vi "Ritter STP Correction.vi"(7 "Meter Type":enum16{"Dry Meter", "Wet Meter"}(ring)=enum."Wet Meter", 8 "error in":errorcluster, 10 "Inficon Data Output":T2, 11 "Ritter Data":T1) -> (0 "error out":errorcluster, 3 "Ritter Data Output":T1)   [LabVIEW 2023]
uses:
  Drivers/Ritter Gas Meter/Type Definitions/Ritter Data.ctl
  Drivers/Inficon Fusion Micro GC/Type Definitions/Inficon Data.ctl
panel:
  # "Natural Gas"
  # "Propane"
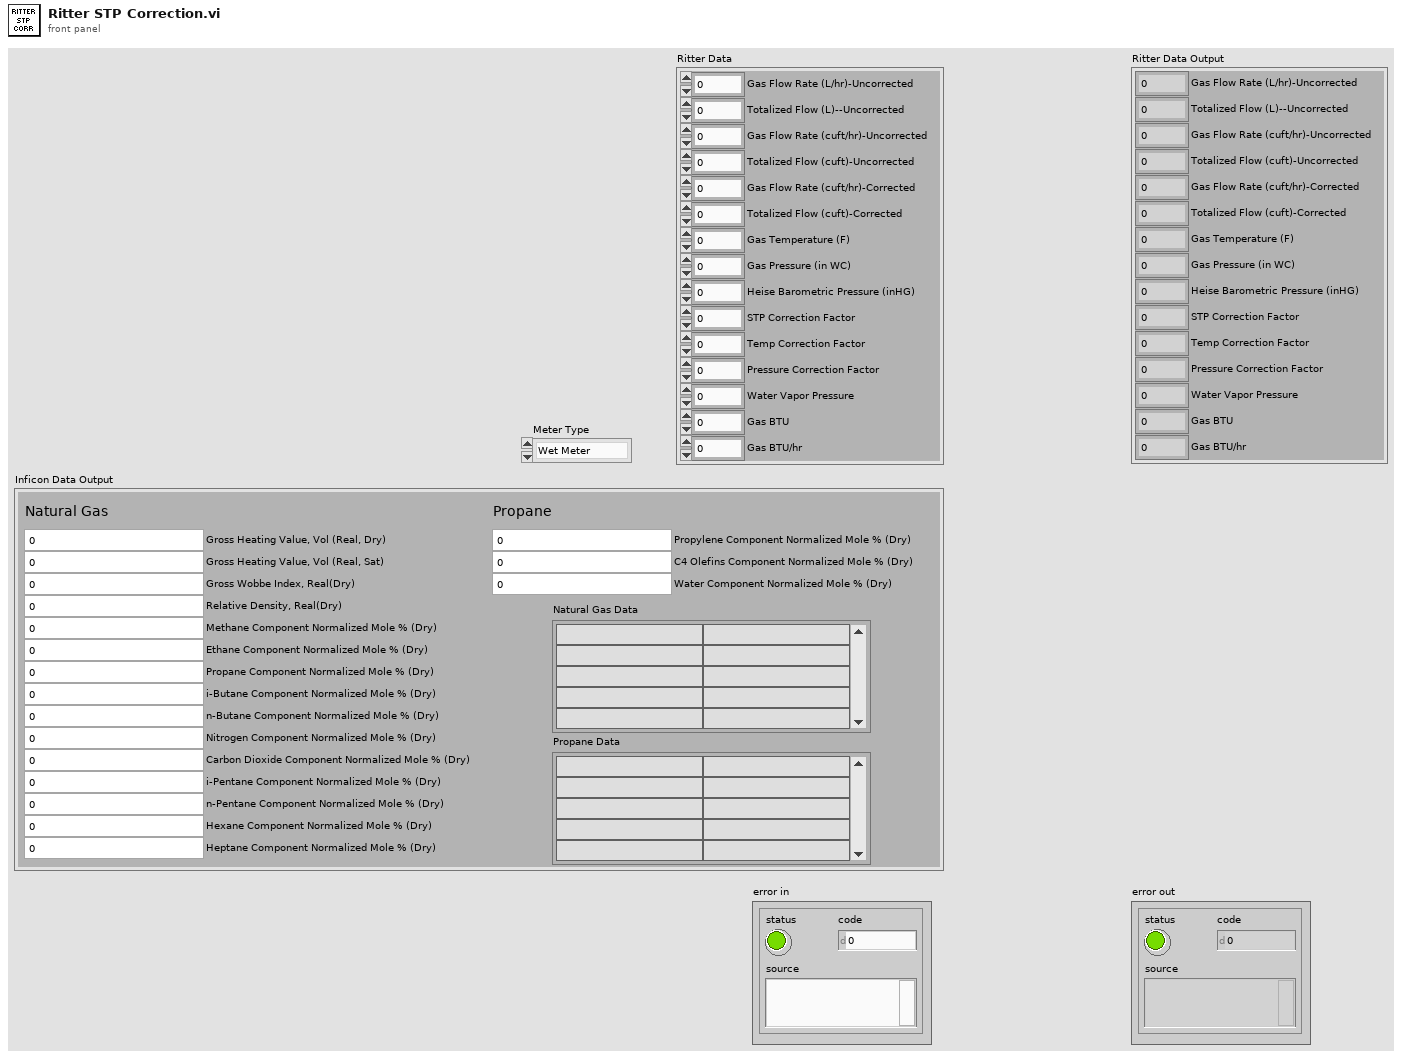
[diagram p1: front panel]
types:
  T1 = typedef "Ritter Data.ctl" = cluster{"Gas Flow Rate (L/hr)-Uncorrected":dbl, "Totalized Flow (L)--Uncorrected":dbl, "Gas Flow Rate (cuft/hr)-Uncorrected":dbl, "Totalized Flow (cuft)-Uncorrected":dbl, "Gas Temperature (F)":dbl, "Gas Pressure (in WC)":dbl, "Heise Barometric Pressure (inHG)":dbl, "STP Correction Factor":dbl, "Temp Correction Factor":dbl, "Pressure Correction Factor":dbl, "Water Vapor Pressure":dbl, "Gas Flow Rate (cuft/hr)-Corrected":dbl, "Totalized Flow (cuft)-Corrected":dbl, "Gas BTU":dbl, "Gas BTU/hr":dbl}
  T2 = typedef "Inficon Data.ctl" = cluster{"Gross Heating Value, Vol (Real, Dry)":dbl, "Nitrogen Component Normalized Mole % (Dry)":dbl, "Methane Component Normalized Mole % (Dry)":dbl, "Carbon Dioxide Component Normalized Mole % (Dry)":dbl, "Ethane Component Normalized Mole % (Dry)":dbl, "Propane Component Normalized Mole % (Dry)":dbl, "i-Pentane Component Normalized Mole % (Dry)":dbl, "i-Butane Component Normalized Mole % (Dry)":dbl, "n-Butane Component Normalized Mole % (Dry)":dbl, "n-Pentane Component Normalized Mole % (Dry)":dbl, "Hexane Component Normalized Mole % (Dry)":dbl, "Heptane Component Normalized Mole % (Dry)":dbl, "Gross Wobbe Index, Real(Dry)":dbl, "Relative Density, Real(Dry)":dbl, "Propylene Component Normalized Mole % (Dry)":dbl, "C4 Olefins Component Normalized Mole % (Dry)":dbl, "Water Component Normalized Mole % (Dry)":dbl, "Gross Heating Value, Vol (Real, Sat)":dbl, "Natural Gas Data":string[][], "Propane Data":string[][]}
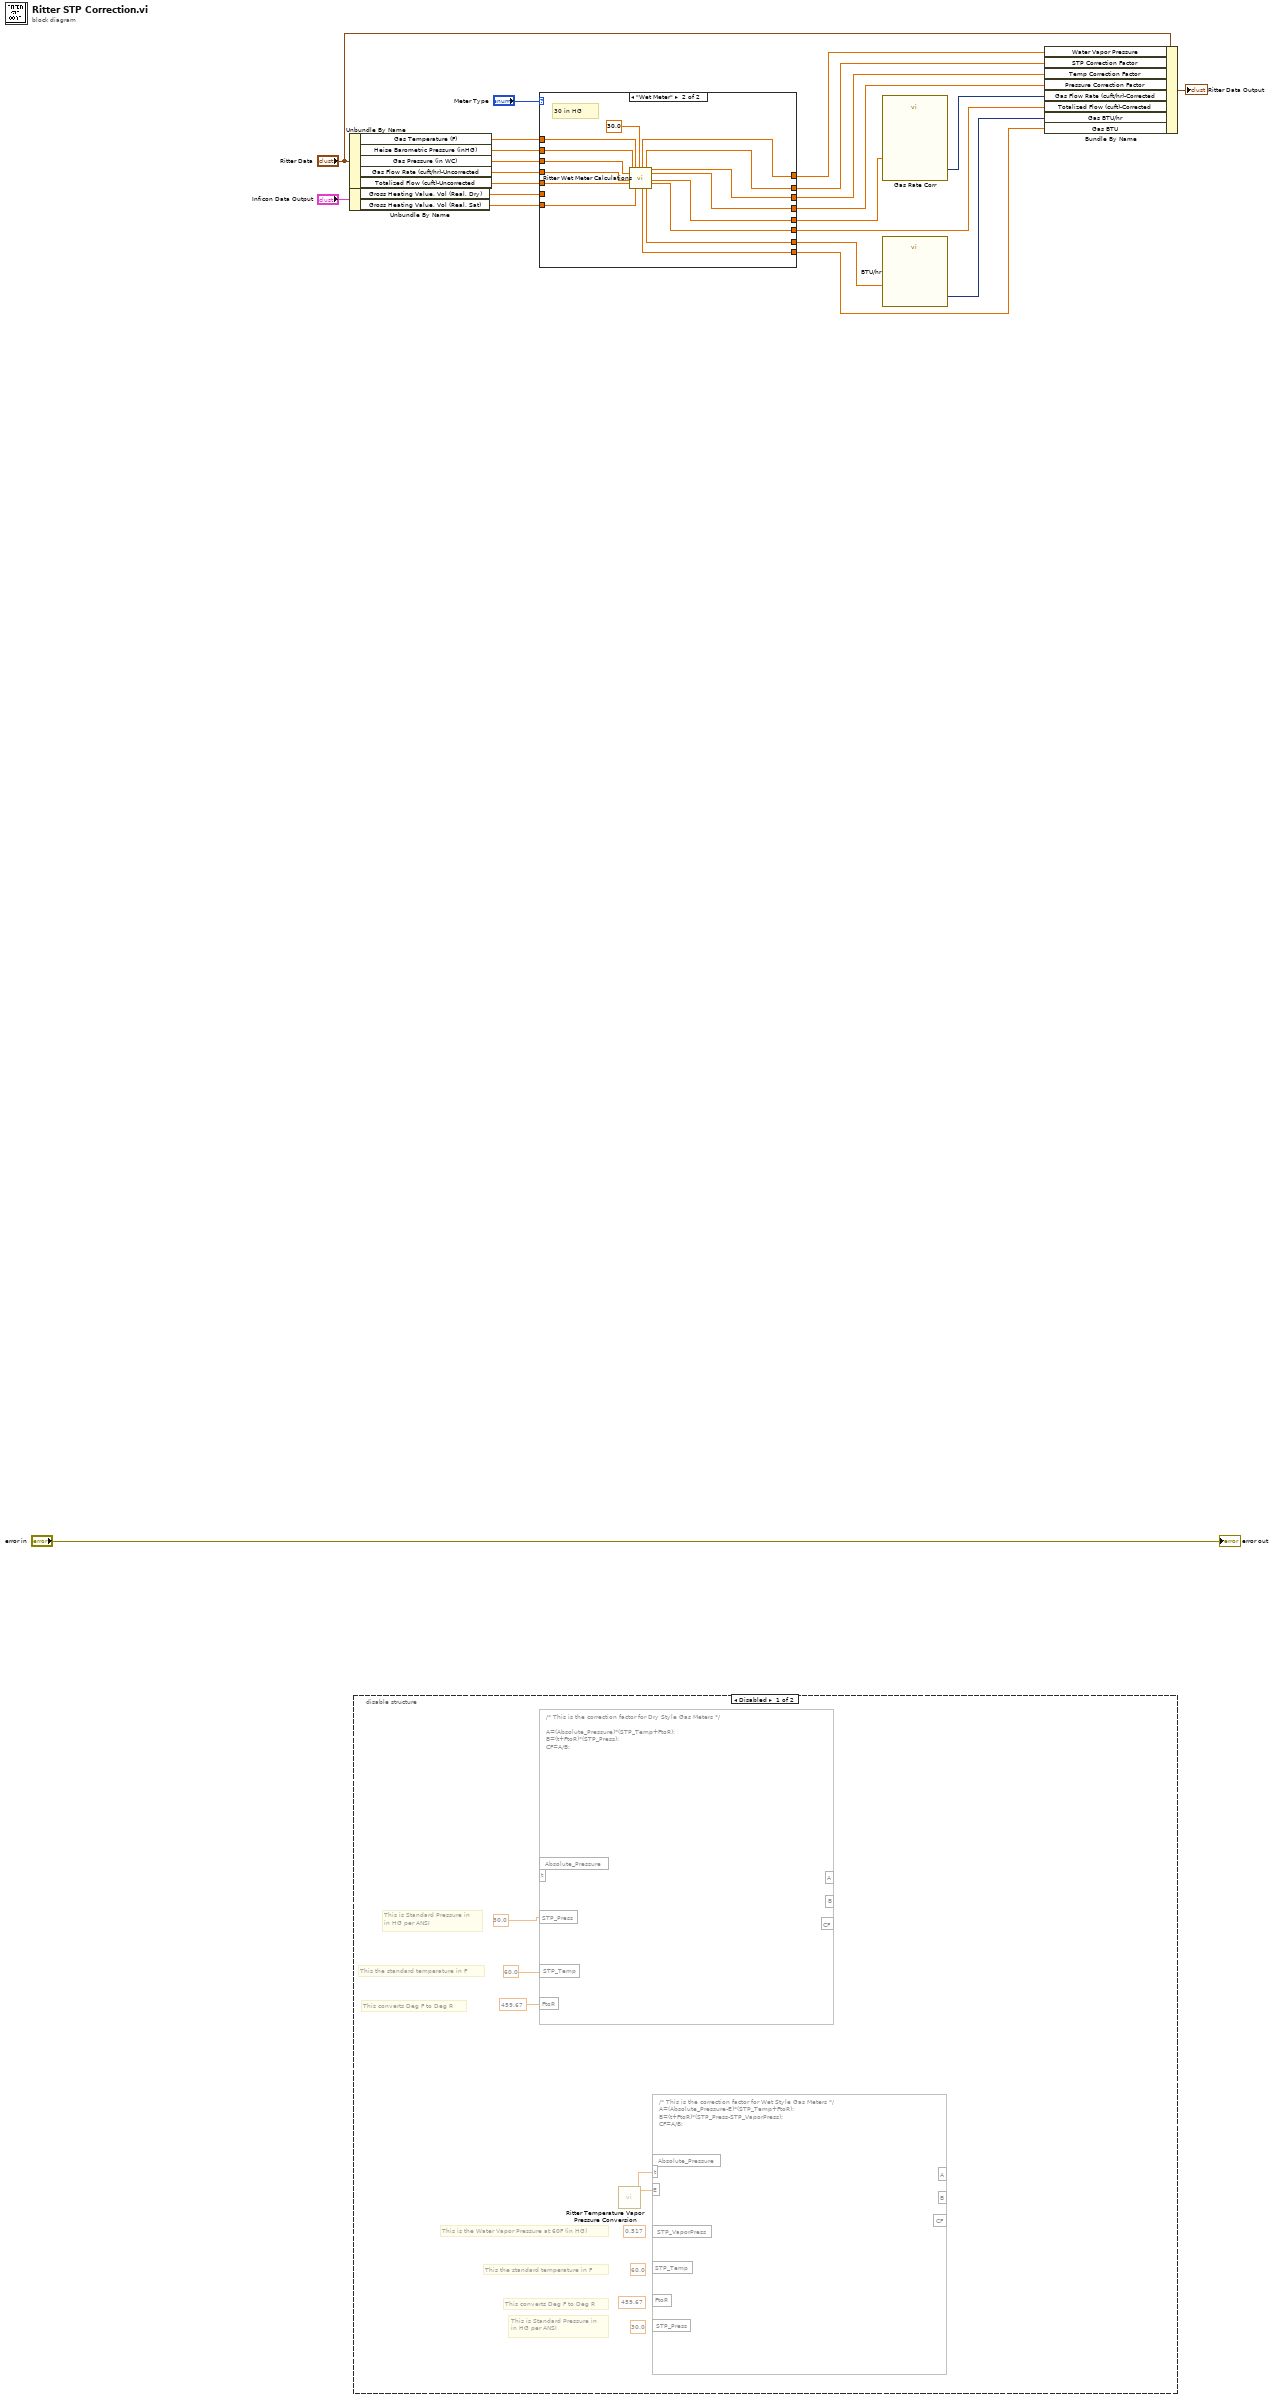
[diagram p0: block diagram]
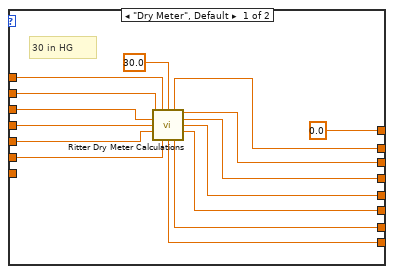
[diagram p3: hidden frame]
diagram:
  n1 = Unbundle By Name("Ritter Data") -> ("Gas Temperature (F)"=w17:dbl, "Heise Barometric Pressure (inHG)"=w16:dbl, "Gas Pressure (in WC)"=w15:dbl, "Gas Flow Rate (cuft/hr)-Uncorrected"=w14:dbl, "Totalized Flow (cuft)-Uncorrected"=w13:dbl)
  n2 = Unbundle By Name("Inficon Data Output") -> ("Gross Heating Value, Vol (Real, Dry)"=w12:dbl, "Gross Heating Value, Vol (Real, Sat)"=w11:dbl)
  n3 = disable-structure shown="Disabled" {
    frame Disabled {
      (unwired) 459.67 ("input variable")
      (unwired) 60.0 ("input variable")
      (unwired) 30.0 ("input variable")
      (unwired) 0.517 ("input variable")
      # "This converts Deg F to Deg R"
      # "This the standard temperature in F"
      # "This is Standard Pressure in\nin HG per ANSI"
      # "This is the Water Vapor Pressure at 60F (in HG)"
      # "This converts Deg F to Deg R"
      # "This the standard temperature in F"
      # "This is Standard Pressure in\nin HG per ANSI"
      n4 = formula code="/* This is the correction factor for Dry Style Gas Meters */\n\nA=(Absolute_Pressure)*(STP_Temp+FtoR);\nB=(t+FtoR)*(STP_Press);\nCF=A/B;"("STP_Press"=30.0 ("input variable"), "STP_Temp"=60.0 ("input variable"), "FtoR"=459.67 ("input variable")) -> ()  [unwired: 2 in, 3 out]
      n5 = call "Ritter Temperature Vapor Pressure Conversion.vi"() -> ("Water Vapor Pressure (in HG)"=w24:dbl, "Temperature Value"=w23:dbl)  [unwired: 9 in, 1 out]
      n6 = formula code="/* This is the correction factor for Wet Style Gas Meters */\nA=(Absolute_Pressure-E)*(STP_Temp+FtoR);\nB=(t+FtoR)*(STP_Press-STP_VaporPress);\nCF=A/B;"("E"=w24, "t"=w23) -> ()  [unwired: 5 in, 3 out]
    }
    frame Enabled {
    }
  }
  n7 = case shown="\"Wet Meter\"" "Meter Type" {
    tunnel: [w40 w54] -> w8
    tunnel: w17 -> [w39 w57]
    tunnel: w16 -> [w42 w56]
    tunnel: w15 -> [w41 w55]
    tunnel: [w38 w53] -> w7
    tunnel: [w37 w52] -> w6
    tunnel: [0.0 ("E") w51] -> w9
    tunnel: w14 -> [w35 w50]
    tunnel: w13 -> [w34 w49]
    tunnel: [w33 w48] -> w19
    tunnel: [w32 w47] -> w4
    tunnel: w12 -> [w31 _]
    tunnel: [w30 w46] -> w20
    tunnel: [w29 w45] -> w1
    tunnel: w11 -> [_ w44]
    frame "Dry Meter", Default {
      # "30 in HG"
      n8 = call "Ritter Dry Meter Calculations.vi"("Heise Barometric Pressure (inHG)"=w42, "Gas Temperature (F)"=w39, "standardPressure (in HG)"=30.0, "Gas Pressure (in WC)"=w41, "Gas Flow Rate (cuft/hr)-Uncorrected"=w35, "Totalized Flow (cuft)-Uncorrected"=w34, "Gross Heating Value, Vol (Real, Dry)"=w31) -> ("CFdry"=w40:dbl, "tempCorrectionFactor"=w38:dbl, "pressureCorrectionFactor"=w37:dbl, "gasFlowRate"=w33:dbl, "gasVolume"=w32:dbl, "btuEnergy"=w29:dbl, "btuRate"=w30:dbl)  [unwired: 1 in, 1 out]
    }
    frame "Wet Meter" {
      # "30 in HG"
      n9 = call "Ritter Wet Meter Calculations.vi"("Heise Barometric Pressure (inHG)"=w56, "Gas Pressure (in WC)"=w55, "Gas Flow Rate (cuft/hr)-Uncorrected"=w50, "Totalized Flow (cuft)-Uncorrected"=w49, "Gas Temperature (F)"=w57, "Gross Heating Value, Vol (Real, Sat)"=w44, "standardPressure (in HG)"=30.0) -> ("E"=w51:dbl, "btuEnergy"=w45:dbl, "CFsat"=w54:dbl, "btuRate"=w46:dbl, "tempCorrectionFactor"=w53:dbl, "pressureCorrectionFactor"=w52:dbl, "gasFlowRate"=w48:dbl, "gasVolume"=w47:dbl)  [unwired: 4 in, 1 out]
    }
  }
  n10 = call "Gas Rate Corr"("Signal"=w19) -> ("Filtered Signal"=w5:dynamicdata)  [unwired: 9 in, 1 out]
  n11 = call "BTU/hr"("Signal"=w20) -> ("Filtered Signal"=w2:dynamicdata)  [unwired: 9 in, 1 out]
  n12 = Bundle By Name(cluster="Ritter Data", "Water Vapor Pressure"=w9, "STP Correction Factor"=w8, "Temp Correction Factor"=w7, "Pressure Correction Factor"=w6, "Gas Flow Rate (cuft/hr)-Corrected"=w5, "Totalized Flow (cuft)-Corrected"=w4, "Gas BTU/hr"=w2, "Gas BTU"=w1) -> (→"Ritter Data Output":T1)
  "error out" <- "error in"
